vi "Eat.vi"(8 "error in (no error)":errorcluster, 10 "String":string, 11 "Sheep in":refnum<class "Sheep.lvclass">) -> (0 "error out":errorcluster, 2 "String 2":string, 3 "Sheep out":refnum<class "Sheep.lvclass">)   [LabVIEW 2018, in "Sheep.lvclass"]
uses:
  Sheep.lvclass
  animal/Animal.lvclass
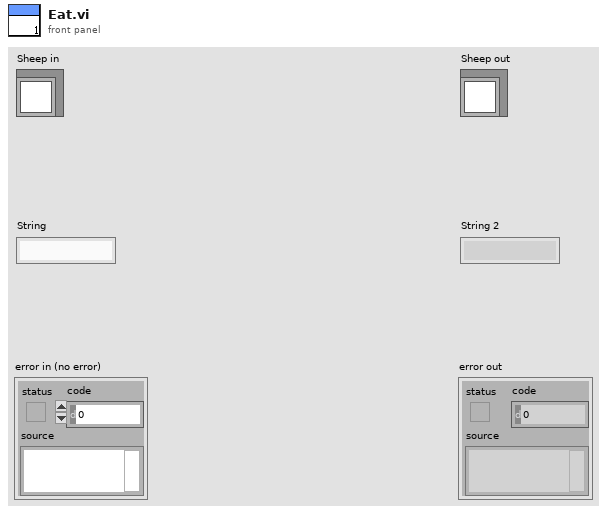
[diagram p1: front panel]
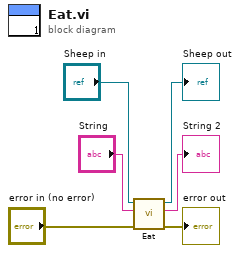
[diagram p0: block diagram]
diagram:
  n1 = call-parent "Eat.vi"("error in (no error)"="error in (no error)", "String"="String", "Animal in"="Sheep in") -> ("error out"=→"error out":errorcluster, "String 2"=→"String 2":string, "Animal out"=→"Sheep out":refnum<class "Sheep.lvclass">)  [unwired: 6 in]
